vi "Smooth Background WFRM DBL.vi"(7 "Type":T1(ring)=enum."Bandpass", 8 "Error In":errorcluster, 9 "HP F":dbl format="%#_6p", 10 "LP  F":dbl=0.001 format="%#_6p", 11 "Data":waveform(dbl)) -> (0 "Error Out":errorcluster, 3 "Data out":waveform(dbl))   [LabVIEW 2016]
uses:
  <vilib>/measure/NI_MAPro.lvlib
  <vilib>/Analysis/3filter.llb/Filter Structure Type.ctl
  <vilib>/Analysis/NI_AALBase.lvlib
  <vilib>/measure/macond.llb/IIR Filter for 1 Chan.vi
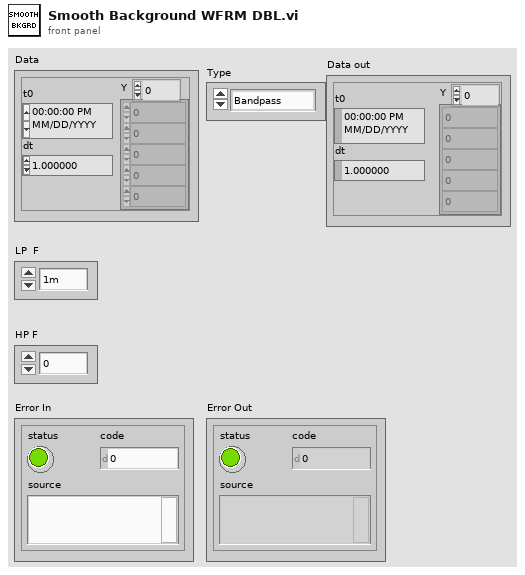
[diagram p1: front panel]
types:
  T1 = enum16{"Lowpass", "Highpass", "Bandpass", "Bandstop"}
  T2 = typedef "NI_AALBase.lvlib/Filter Structure Type.ctl" = u16
  T3 = cluster{"Topology":enum16{"Off", "Butterworth", "Chebyshev", "Inverse Chebyshev", "Elliptic", "Bessel"}, "Type":enum16{"Lowpass", "Highpass", "Bandpass", "Bandstop"}, "Order":i32, "Lower Fc":dbl, "Upper Fc":dbl, "PB Ripple":dbl, "SB Attenuation":dbl}
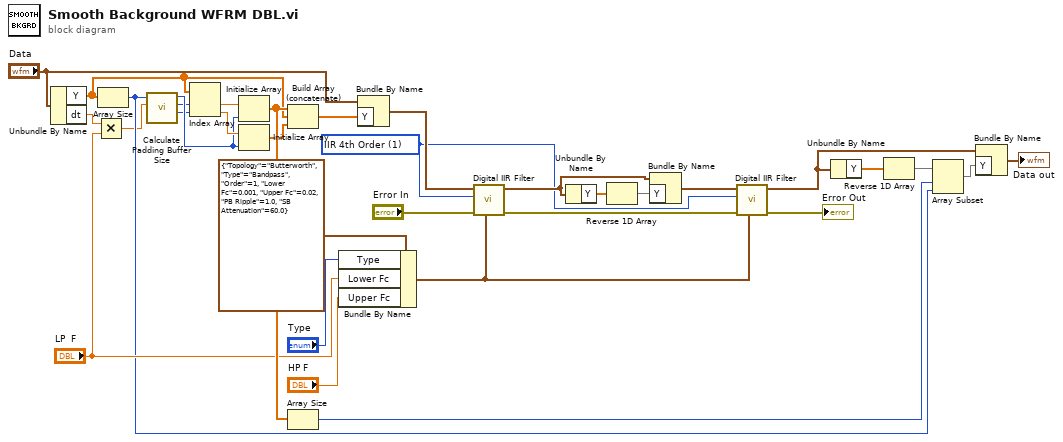
[diagram p0: block diagram]
diagram:
  w21 = T2 1 items=["IIR 2nd Order"=0, "IIR 4th Order"=1, "Auto Select"=10] ("filter structure option")
  n1 = Unbundle By Name("Data") -> ("Y"=w12:dbl[], "dt"=w10:dbl)
  n2 = Multiply(x=w10, y="LP  F") -> (x*y=w3:dbl)
  n3 = Array Size(array=w12) -> (size(s)=w5:i32)
  n4 = call "Calculate Padding Buffer Size.vi"("LP  F"=w3, "Array size"=w5) -> ("Last element"=w1:i32, "First element"=w2:i32, "Buffer size"=w4:i32)  [unwired: 7 in]
  n5 = Index Array(array=w12, index #1=w2, index #2=w1) -> (element #1=w31:dbl, element #2=w16:dbl)
  n6 = Initialize Array(w31, w4) -> (w33:dbl[])
  n7 = Initialize Array(w16, w4) -> (w15:dbl[])
  n8 = Build Array (concatenate)(w33, w12, w15) -> (w32:dbl[])
  n9 = Array Size(array=w33) -> (size(s)=w17:i32)
  n10 = Bundle By Name(cluster=T3 {"Topology"=enum."Butterworth", "Type"=enum."Bandpass", "Order"=1, "Lower Fc"=0.001, "Upper Fc"=0.02, "PB Ripple"=1.0, "SB Attenuation"=60.0} ("IIR filter specifications"), "Type"="Type", "Lower Fc"="LP  F", "Upper Fc"="HP F") -> (w22:T3)
  n11 = Bundle By Name(cluster="Data", "Y"=w32) -> (w30:waveform(dbl))
  n12 = call-poly <vilib>:"Digital IIR Filter.vi"("IIR filter specifications"=w22, "error in (no error)"="Error In", "filter structure option"=w21, "signal in"=w30) -> ("error out"=w20:errorcluster, "signal out"=w25:waveform(dbl))  [unwired: 5 in, 1 out]
  n13 = Unbundle By Name(w25) -> ("Y"=w26:dbl[])
  n14 = Reverse 1D Array(array=w26) -> (reversed array=w24:dbl[])
  n15 = Bundle By Name(cluster=w25, "Y"=w24) -> (w23:waveform(dbl))
  n16 = call-poly <vilib>:"Digital IIR Filter.vi"("IIR filter specifications"=w22, "error in (no error)"=w20, "filter structure option"=w21, "signal in"=w23) -> ("error out"=→"Error Out":errorcluster, "signal out"=w9:waveform(dbl))  [unwired: 5 in, 1 out]
  n17 = Unbundle By Name(w9) -> ("Y"=w19:dbl[])
  n18 = Reverse 1D Array(array=w19) -> (reversed array=w18:dbl[])
  n19 = Array Subset(array=w18, index=w17, length=w5) -> (w7:dbl[])
  n20 = Bundle By Name(cluster=w9, "Y"=w7) -> (→"Data out":waveform(dbl))
